vi "GenerateFilenames_IOS.vi"(11 "path":path) -> (0 "TDMS Path":path, 1 "Dalsa Path":path, 2 "Basler Path":path, 3 "WebCam Path":path, 4 "Analog file name":string="F:\\Data\\130725_14_35_2625", 5 "Basler2 Path":path)   [LabVIEW 2017]
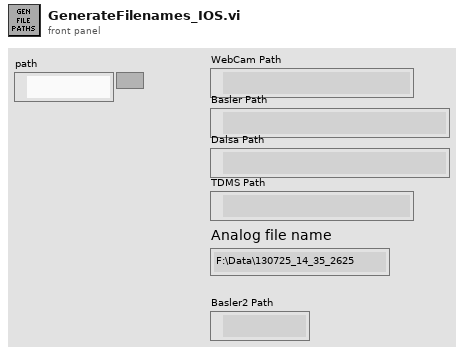
[diagram p1: front panel]
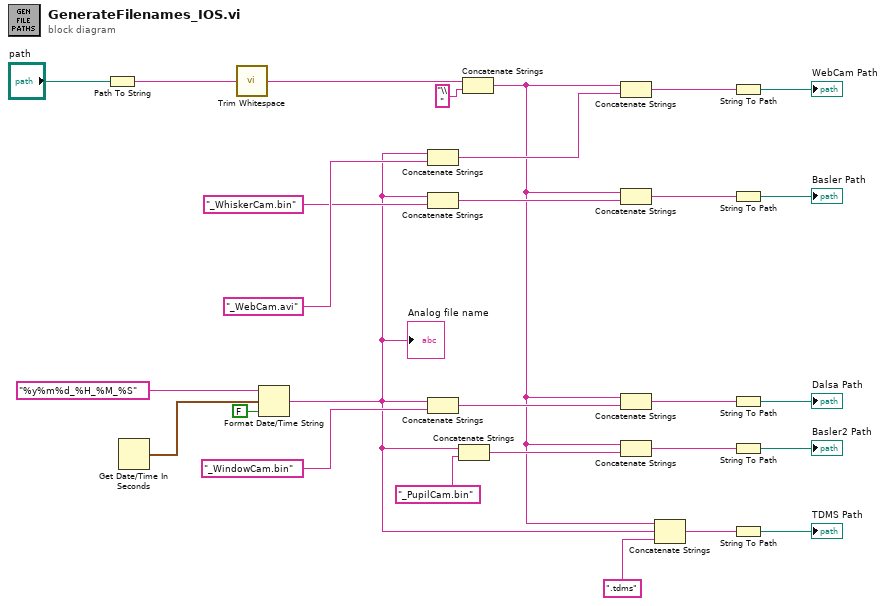
[diagram p0: block diagram]
diagram:
  n1 = Path To String(path="path") -> (string=w10:string)
  n2 = Get Date/Time In Seconds() -> (seconds since 1Jan1904=w27:timestamp)
  n3 = call <vilib>:"Trim Whitespace.vi"("string"=w10) -> ("trimmed string"=w8:string)  [unwired: 1 in]
  n4 = Format Date/Time String(time format string (%c)="%y%m%d_%H_%M_%S", seconds (now)=w27, UTC format=FALSE) -> (date/time string=w2:string)
  "Analog file name" <- w2
  n5 = Concatenate Strings(w2, "_WebCam.avi") -> (w25:string)
  n6 = Concatenate Strings(w2, "_WhiskerCam.bin" ("string")) -> (w19:string)
  n7 = Concatenate Strings(w2, "_WindowCam.bin") -> (w23:string)
  n8 = Concatenate Strings(w2, "_PupilCam.bin" ("string")) -> (w5:string)
  n9 = Concatenate Strings(w8, "\\" ("string")) -> (w1:string)
  n10 = Concatenate Strings(w1, w25) -> (w21:string)
  n11 = Concatenate Strings(w1, w19) -> (w18:string)
  n12 = Concatenate Strings(w1, w23) -> (w22:string)
  n13 = Concatenate Strings(w1, w5) -> (w4:string)
  n14 = Concatenate Strings(w1, w2, ".tdms" ("string")) -> (w11:string)
  n15 = String To Path(string=w21) -> (path=→"WebCam Path":path)
  n16 = String To Path(string=w18) -> (path=→"Basler Path":path)
  n17 = String To Path(string=w22) -> (path=→"Dalsa Path":path)
  n18 = String To Path(string=w4) -> (path=→"Basler2 Path":path)
  n19 = String To Path(string=w11) -> (path=→"TDMS Path":path)
